vi "FullBackProp_multiple.vi"(4 "Target":dbl[](array[numeric]), 5 "appended array":dbl[](array[numeric]), 6 "Array 3":dbl[](array[numeric]), 7 "Array 4":dbl[](array[numeric]), 8 "dE_dNET 2":dbl[](array[numeric]), 9 "dE_dNET":dbl[](array[numeric]), 10 "Array 2":dbl[](array[numeric]), 11 "Array":dbl[](array[numeric])) -> (2 "w+":fxp<+/-,64,32>[](array[numeric]), 3 "w+ 2":fxp<+/-,64,32>[](array[numeric]))   [LabVIEW 2014]
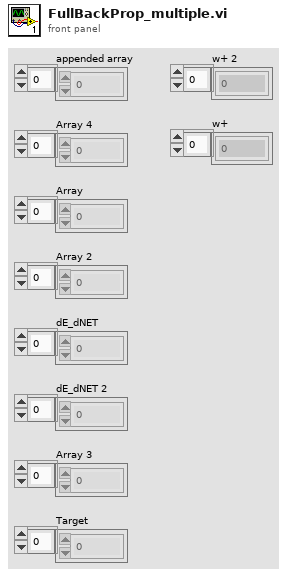
[diagram p1: front panel]
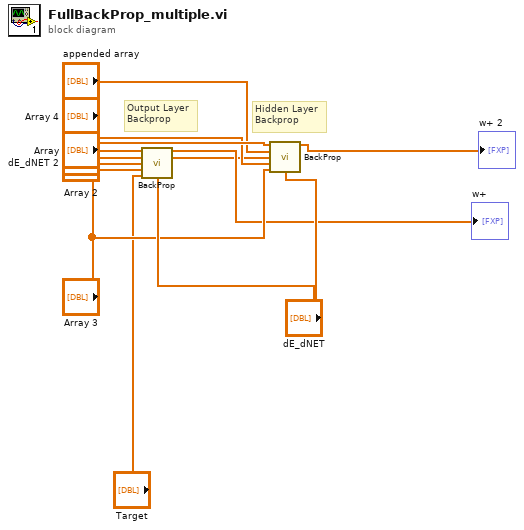
[diagram p0: block diagram]
diagram:
  # "Hidden Layer\nBackprop"
  # "Output Layer\nBackprop"
  n1 = call "BackProp.vi"("Current Layer"="Array", "Previous Layer"="Array 2", "NetError"="dE_dNET 2", "weights"="Array 3", "PreviousWeights"="Target", "Target"="dE_dNET") -> ("w+"=→"w+":dbl[], "dE_dNET"=w1:dbl[])  [unwired: 8 in]
  n2 = call "BackProp.vi"("Current Layer"="Array 2", "Previous Layer"="appended array", "NetError"=w1, "weights"="Array 4", "PreviousWeights"="Array 3", "Target"="dE_dNET") -> ("w+"=→"w+ 2":dbl[])  [unwired: 8 in, 1 out]
